vi "Read value.vi"(8 "error in (no error)":errorcluster, 11 "AISAS Mech in":refnum<class "AISAS Mech.lvclass">) -> (0 "error out":errorcluster, 1 "Rotation":T2 format="%.1f", 2 "Focus":T4=70.0 min=15.0 max=155.0 format="%.2f", 3 "Diffuser":T3=enum."In Beam", 4 "Motor":T1, 5 "Value (String)":string, 7 "Motor (String)":string)   [LabVIEW 2014, in "AISAS Mech.lvclass"]
uses:
  AISAS Mech.lvclass
  Controls/focus.ctl
  Controls/Diffuser.ctl
  Controls/Rotation.ctl
  Controls/motor.ctl
  AISAS Mech.lvclass/AISAS Mech.ctl
  motor/AISAS motor.lvclass/AISAS motor.ctl
  motor/AISAS motor.lvclass
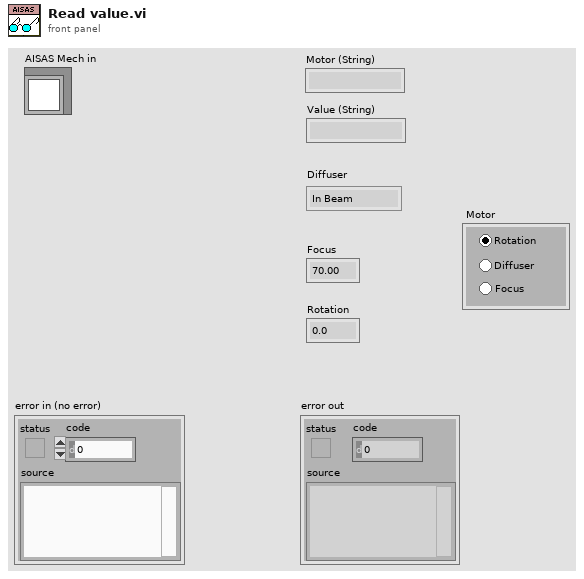
[diagram p1: front panel]
types:
  T1 = typedef "motor.ctl" = enum32{"Rotation", "Diffuser ", "Focus"}
  T2 = typedef "Rotation.ctl" = dbl
  T3 = typedef "Diffuser.ctl" = enum16{"Out of Beam", "In Beam"}
  T4 = typedef "focus.ctl" = dbl
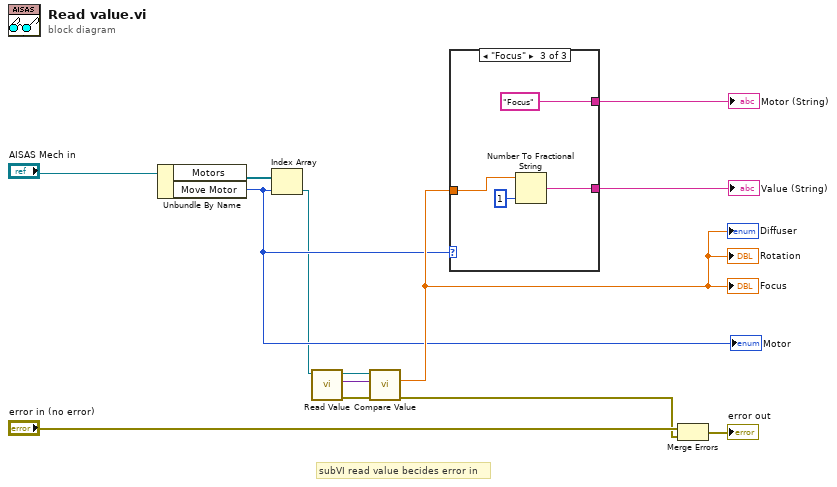
[diagram p0: block diagram]
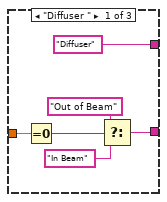
[diagram p2: hidden frame]
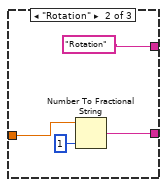
[diagram p3: hidden frame]
diagram:
  # "subVI read value becides error in"
  n1 = Unbundle By Name("AISAS Mech in") -> ("Motors"=w8:refnum<class "AISAS motor.lvclass">[], "Move Motor"=w9:T1)
  "Motor" <- w9
  n2 = Index Array(array=w8, index=w9) -> (element=w7:refnum<class "AISAS motor.lvclass">)
  n3 = call "Read Value.vi"("AISAS motor in"=w7) -> ("error out"=w4:errorcluster, "Value"=w5:variant, "AISAS motor out"=w6:refnum<class "AISAS motor.lvclass">)  [unwired: 8 in]
  n4 = call "Compare Value.vi"("error in (no error)"=w4, "new Value"=w5, "AISAS motor in"=w6) -> ("error out"=w2:errorcluster, "old value"=w12:dbl)  [unwired: 3 in, 4 out]
  "Focus" <- w12
  "Diffuser" <- w12
  "Rotation" <- w12
  n5 = case shown="\"Focus\"" w9 {
    tunnel: ["Diffuser" "Rotation" "Focus"] -> w10
    tunnel: w12 -> [w14 w20 w25]
    tunnel: [w15 w21 w24] -> w11
    frame "Diffuser " {
      n6 = Equal To 0?(x=w14) -> (x = 0?=w18:bool)
      n7 = Select(t="Out of Beam", s=w18, f="In Beam") -> (s? t:f=w15:string)
    }
    frame "Rotation" {
      n8 = Number To Fractional String(number=w20, precision (6)=i16 1) -> (F-format string=w21:string)  [unwired: 2 in]
    }
    frame "Focus" {
      n9 = Number To Fractional String(number=w25, precision (6)=i16 1) -> (F-format string=w24:string)  [unwired: 2 in]
    }
  }
  "Value (String)" <- w11
  "Motor (String)" <- w10
  n10 = Merge Errors("error in (no error)", w2) -> (→"error out":errorcluster)
